vi "toJSON.vi"(8 "error in (no error)":errorcluster, 11 "tBSONArray in":refnum<class "tBSONArray.lvclass">) -> (0 "error out":errorcluster, 2 "JSON":string, 3 "tBSONArray out":refnum<class "tBSONArray.lvclass">)   [LabVIEW 2013, in "BSON.lvlib" / "tBSONArray.lvclass"]
uses:
  tBSONArray.lvclass
  tBSONElement/tBSONElement.lvclass
  getValue.vi
  <vilib>/regexp/Match Regular Expression.xnode
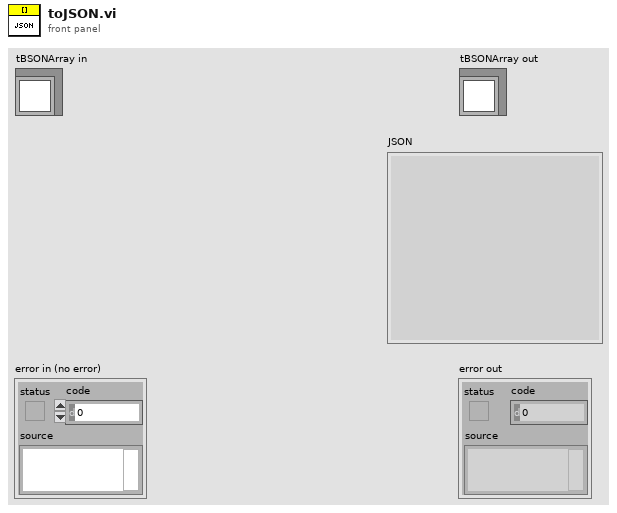
[diagram p1: front panel]
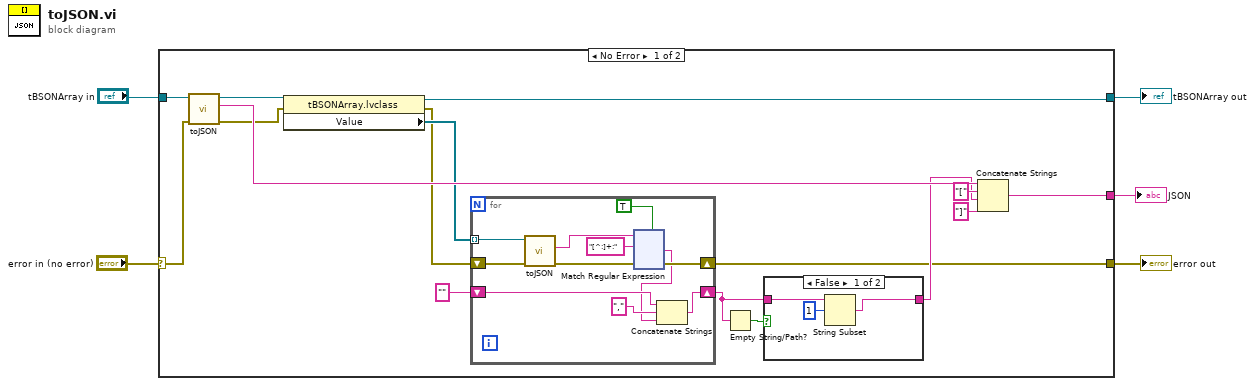
[diagram p0: block diagram]
diagram:
  n1 = case shown="No Error" "error in (no error)" {
    selector: "error in (no error)" -> [w20 w149]
    tunnel: "tBSONArray in" -> [w21 w148]
    tunnel: [w16 _] -> w3
    tunnel: [w13 w148] -> w2
    tunnel: [w6 w149] -> w1
    frame No Error {
      n2 = call-parent "toJSON.vi"("error in (no error)"=w20, "tBSONElement in"=w21) -> ("error out"=w14:errorcluster, "JSON"=w19:string, "tBSONElement out"=w15:refnum<class "tBSONArray.lvclass">)  [unwired: 7 in]
      n3 = property class="tBSONArray.lvclass"(reference=w15, error in=w14) -> (reference out=w13:refnum<class "tBSONArray.lvclass">, error out=w11:errorcluster, "Value"=w12:refnum<class "tBSONElement.lvclass">[])
      n4 = for {
        tunnel: w12 -> [w36] mode=indexing
        shift-right: [w34] -> w8
        shift-left: "" -> [w32]
        shift-right: [w28] -> w6
        shift-left: w11 -> [w35]
        n5 = call-dynamic "toJSON.vi"("error in (no error)"=w35, "tBSONElement in"=w36) -> ("error out"=w31:errorcluster, "JSON"=w30:string)  [unwired: 7 in, 1 out]
        n6 = xnode "Match Regular Expression"("input string"=w30, "regular expression"="[^:]+:", "error in"=w31, "multiline? (F)"=TRUE) -> ("after match"=w26:string, "error out"=w28:errorcluster)  [unwired: 2 in, 3 out]
        n7 = Concatenate Strings(w32, "," ("string"), w26) -> (w34:string)
      }
      n8 = Empty String/Path?(string/path=w8) -> (empty?=w9:bool)
      n9 = case shown="False" w9 {
        tunnel: w8 -> [w24 w25]
        tunnel: [w22 w25] -> w7
        frame False {
          n10 = String Subset(string=w24, offset (0)=1) -> (substring=w22:string)  [unwired: 1 in]
        }
        frame True {
        }
      }
      n11 = Concatenate Strings(w19, "[" ("string"), w7, "]" ("string")) -> (w16:string)
    }
    frame Error {
    }
  }
  "error out" <- w1
  "tBSONArray out" <- w2
  "JSON" <- w3
